vi "DSF.UDP.Transfer.Get Port.vi"(8 "error in (no error)":errorcluster, 11 "UDP Transfer in":refnum<class "DSF.Plugin.UDP.Configuration.Transfer.lvclass">) -> (0 "error out":errorcluster, 2 "Port":u16, 3 "UDP Transfer out":refnum<class "DSF.Plugin.UDP.Configuration.Transfer.lvclass">)   [LabVIEW 2016, in "DSF.Plugin.UDP.Configuration.Transfer.lvclass"]
uses:
  DSF.Plugin.UDP.Configuration.Transfer.lvclass
  DSF.Plugin.UDP.Configuration.Transfer.lvclass/DSF.Plugin.UDP.Configuration.Transfer.ctl
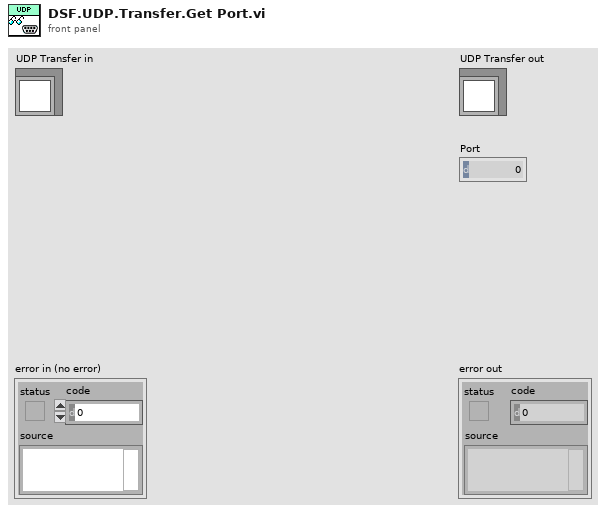
[diagram p1: front panel]
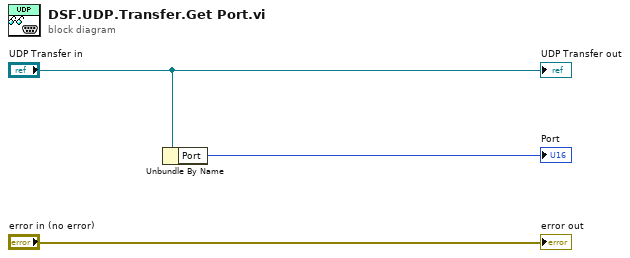
[diagram p0: block diagram]
diagram:
  n1 = Unbundle By Name("UDP Transfer in") -> ("Port"=→"Port":u16)
  "error out" <- "error in (no error)"
  "UDP Transfer out" <- "UDP Transfer in"
